vi "Fix XML.vi"() -> ()   [LabVIEW 2013]
uses:
  <vilib>/xml/Close Reference(Node).vi
  <resource>/objmgr/DOMUserDefRef.rc
  <vilib>/xml/NI_XML.lvlib
panel:
  in  "Destination XML File Path":path
  in  "Default Values":string="<?xml version=\"1.0\" encoding=\"utf-8\"?>\n<ArrayOfGsSequenceUnit xmlns:xsi=\"http://www.w3.org/2001/XMLSchema-instance\" xmlns:xsd=\"http://www.w3.org/2001/XMLSchema\">\n<gsSequenceUnit>\n    <AutoNumberTag />\n    <TimingSettings>\n      <Settings>\n        <MassSpecTriggerType>None</MassSpecTriggerType>\n        <MassSpecTriggerType>None</MassSpecTriggerType>\n        <MassSpecTriggerType>None</MassSpecTriggerType>\n        <MassSpecTriggerType>None</MassSpecTriggerType>\n        <MassSpecTriggerType>Pulse</MassSpecTriggerType>\n        <MassSpecTriggerType>Pulse</MassSpecTriggerType>\n        <MassSpecTriggerType>None</MassSpecTriggerType>\n        <MassSpecTriggerType>None</MassSpecTriggerType>\n      </Settings>\n    </TimingSettings>\n    \n    <DelaySettings>\n      <Settings>\n        <TimingSettingsPair>\n          <Units>s</Units>\n          <Value>27</Value>\n        </TimingSettingsPair>\n        <TimingSettingsPair>\n          <Units>s</Units>\n          <Value>0</Value>\n        </TimingSettingsPair>\n        <TimingSettingsPair>\n          <Units>s</Units>\n          <Value>6.5</Value>\n        </TimingSettingsPair>\n        <TimingSettingsPair>\n          <Units>s</Units>\n          <Value>0</Value>\n        </TimingSettingsPair>\n      </Settings>\n    </DelaySettings>\n\n    <CleaningPointNumShots>0</CleaningPointNumShots>\n    <CleaningPointSpotSizePosition>1</CleaningPointSpotSizePosition>\n    <CleaningPathEnable>false</CleaningPathEnable>\n    <CleaningPathOverlap>50</CleaningPathOverlap>\n    <CleaningPathSpotSizePosition>1</CleaningPathSpotSizePosition>\n    <CleaningPathRepRate>8.00</CleaningPathRepRate>\n    <CleaningPathNumPasses>1</CleaningPathNumPasses>\n    <UseDynamicGasFlows>true</UseDynamicGasFlows>\n    <GasN2Flow>4.0</GasN2Flow>\n    <GasN2Flow_units>ml/min</GasN2Flow_units>\n    <GasHeFlow>950</GasHeFlow>\n    <GasHeFlow_units>ml/min</GasHeFlow_units>\n    <UseDynamicRepRate>false</UseDynamicRepRate>\n    <LaserRepRate>8.00</LaserRepRate>\n    <UseDynamicEnergy>false</UseDynamicEnergy>\n    <LaserEnergy>180</LaserEnergy>\n    <UseDynamicSpotSize>false</UseDynamicSpotSize>\n    <LaserSpotSizePosition>7</LaserSpotSizePosition>\n    <UseDynamicAttenuator>false</UseDynamicAttenuator>\n    <Attenuator>2</Attenuator>\n    <UseDynamicSlitAngle>false</UseDynamicSlitAngle>\n    <RotatingSlitBehaviour>Fixed</RotatingSlitBehaviour>\n    <FixedRotatingSlitAngle>0</FixedRotatingSlitAngle>\n    <TypeEnumerator>0</TypeEnumerator>\n    <ExactStagePointX>12113</ExactStagePointX>\n    <ExactStagePointY>40144</ExactStagePointY>\n    <ExactStagePointZ>0</ExactStagePointZ>\n    <StagePointAblationTime>30.0</StagePointAblationTime>\n    <StagePointAblationTime_units>s</StagePointAblationTime_units>\n    <StatePointAblationShotsOverride>0</StatePointAblationShotsOverride>\n    <StagePathScanSpeed>0</StagePathScanSpeed>\n    <StagePathSplineCurve>false</StagePathSplineCurve>\n    <StageDiscretePointSpacing>0</StageDiscretePointSpacing>\n    <StageDiscreteNumPoints>0</StageDiscreteNumPoints>\n    <StageDiscreteTypeEnum>0</StageDiscreteTypeEnum>\n    <StageDiscreteAblationTime>0</StageDiscreteAblationTime>\n    <StateDiscreteAblationShotsOverride>0</StateDiscreteAblationShotsOverride>\n    <StageGridXSpacing>0</StageGridXSpacing>\n    <StageGridYSpacing>0</StageGridYSpacing>\n    <StageGridAblationTime>0</StageGridAblationTime>\n    <StateGridAblationShotsOverride>0</StateGridAblationShotsOverride>\n    <StageGridAngle>0</StageGridAngle>\n    <StageGridPattern>Raster</StageGridPattern>\n    <StageAreaSpacing>0</StageAreaSpacing>\n    <StageAreaScanSpeed>0</StageAreaScanSpeed>\n    <StageAreaAngle>0</StageAreaAngle>\n    <StageAreaPattern>Raster</StageAreaPattern>\n    <StageAreaEdgeBehaviour>Trace</StageAreaEdgeBehaviour>\n    <Vertices />\n    <_CacheVertixPathLength>0</_CacheVertixPathLength>\n    <Comment>SREF3_1</Comment>\n    <StagePointX>12113</StagePointX>\n    <StagePointY>40144</StagePointY>\n    <StagePointZ>0</StagePointZ>\n  </gsSequenceUnit>\n</ArrayOfGsSequenceUnit>"
  out "error out":errorcluster
  in  "XML File Path":path
  in  "error in (no error)":errorcluster
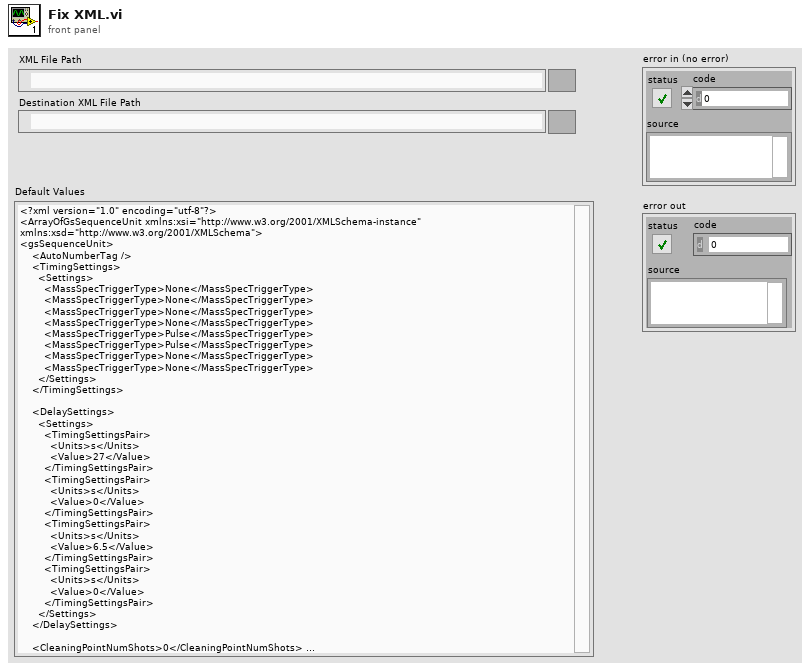
[diagram p1: front panel]
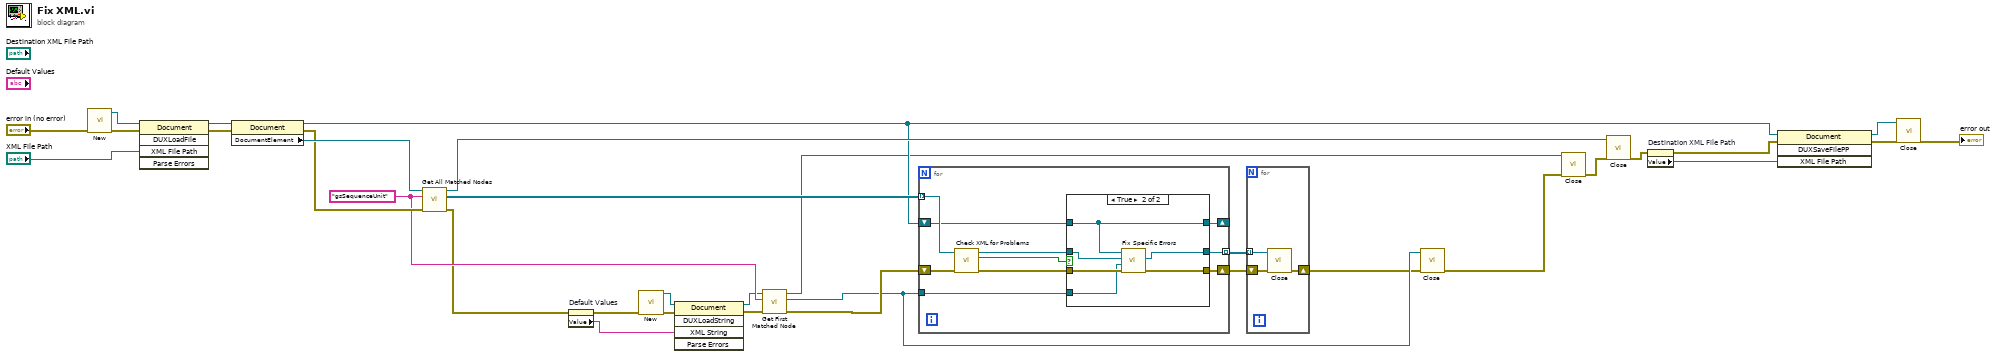
[diagram p0: block diagram]
diagram:
  w21 = "gsSequenceUnit" ("XPath expression")
  n1 = call <vilib>:"New.vi"("error in (no error)"="error in (no error)") -> ("error out"=w32:errorcluster, "DOM document out"=w30:refnum<k20>)  [unwired: 7 in]
  n2 = invoke class="Document" method="DUXLoadFile"(reference=w30, error in=w32, "XML File Path"="XML File Path") -> (reference out=w28:refnum<k20>, error out=w27:errorcluster)  [unwired: 2 in, 3 out]
  n3 = property class="Document"(reference=w28, error in=w27) -> (reference out=w18:refnum<k20>, error out=w24:errorcluster, "DocumentElement"=w29:refnum<k20>)
  n4 = call <vilib>:"Get All Matched Nodes.vi"("error in (no error)"=w24, "XPath expression"=w21, "node in"=w29) -> ("error out"=w2:errorcluster, "node result array"=w23:refnum<k20>[], "node out"=w25:refnum<k20>)  [unwired: 6 in]
  n5 = property on="Default Values" class="Str"(error in=w2) -> (error out=w6:errorcluster, "Value"=w7:string)  [unwired: 1 in, 1 out]
  n6 = call <vilib>:"New.vi"("error in (no error)"=w6) -> ("error out"=w4:errorcluster, "DOM document out"=w5:refnum<k20>)  [unwired: 7 in]
  n7 = invoke class="Document" method="DUXLoadString"(reference=w5, error in=w4, "XML String"=w7) -> (reference out=w3:refnum<k20>, error out=w8:errorcluster)  [unwired: 2 in, 3 out]
  n8 = call <vilib>:"Get First Matched Node.vi"("error in (no error)"=w8, "XPath expression"=w21, "node in"=w3) -> ("error out"=w22:errorcluster, "node result"=w10:refnum<k20>, "node out"=w17:refnum<k20>)  [unwired: 6 in]
  n9 = for {
    tunnel: w23 -> [w42] mode=indexing
    shift-right: [w38] -> w12
    shift-left: w22 -> [w43]
    tunnel: w10 -> [w37]
    shift-right: [w35] -> _
    shift-left: w18 -> [w36]
    tunnel: [w34] -> w11 mode=indexing
    n10 = call "Check XML for Problems.vi"("error in (no error)"=w43, "Node"=w42) -> ("error out"=w39:errorcluster, "Has Problems?"=w41:bool, "Node out"=w40:refnum<k20>)  [unwired: 7 in]
    n11 = case shown="True" w41 {
      tunnel: w40 -> [w44 w48]
      tunnel: w39 -> [w45 w52]
      tunnel: [w45 w51] -> w38
      tunnel: w37 -> [_ w49]
      tunnel: w36 -> [w46 w50]
      tunnel: [w46 w50] -> w35
      tunnel: [w44 w47] -> w34
      frame False {
      }
      frame True {
        n12 = call "Fix Specific Errors.vi"("error in (no error)"=w52, "Good (reference) Node"=w49, "Node to Fix"=w48, "DOM document"=w50) -> ("error out"=w51:errorcluster, "Node to Fix out"=w47:refnum<k20>)  [unwired: 6 in]
      }
    }
  }
  n13 = for {
    shift-right: [w54] -> w1
    shift-left: w12 -> [w55]
    tunnel: w11 -> [w53] mode=indexing
    n14 = call-poly <vilib>:"Close.vi"("error in (no error)"=w55, "node"=w53) -> ("error out"=w54:errorcluster)  [unwired: 7 in]
  }
  n15 = call-poly <vilib>:"Close.vi"("error in (no error)"=w1, "node"=w10) -> ("error out"=w9:errorcluster)  [unwired: 7 in]
  n16 = call-poly <vilib>:"Close.vi"("error in (no error)"=w9, "node"=w17) -> ("error out"=w16:errorcluster)  [unwired: 7 in]
  n17 = call-poly <vilib>:"Close.vi"("error in (no error)"=w16, "node"=w25) -> ("error out"=w15:errorcluster)  [unwired: 7 in]
  n18 = property on="Destination XML File Path" class="Path"(error in=w15) -> (error out=w13:errorcluster, "Value"=w14:path)  [unwired: 1 in, 1 out]
  n19 = invoke class="Document" method="DUXSaveFilePP"(reference=w18, error in=w13, "XML File Path"=w14) -> (reference out=w19:refnum<k20>, error out=w20:errorcluster)  [unwired: 1 in, 2 out]
  n20 = call-poly <vilib>:"Close.vi"("error in (no error)"=w20, "node"=w19) -> ("error out"=→"error out":errorcluster)  [unwired: 7 in]
